vi "Flatten Value.vi"(8 "Error In":errorcluster, 11 "2D String In":refnum<class "2D String.lvclass">) -> (0 "Error Out":errorcluster, 1 "Value":string, 3 "2D String Out":refnum<class "2D String.lvclass">)   [LabVIEW 2017, in "Tree API.lvlib" / "2D String.lvclass"]
doc: "Dynamic dispatch interface for flattening Tree Data classes to string."
uses:
  2D String.lvclass
  Tree Manager/Tree.lvclass
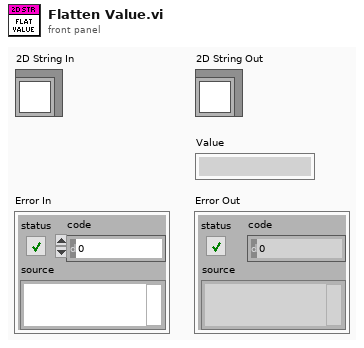
[diagram p1: front panel]
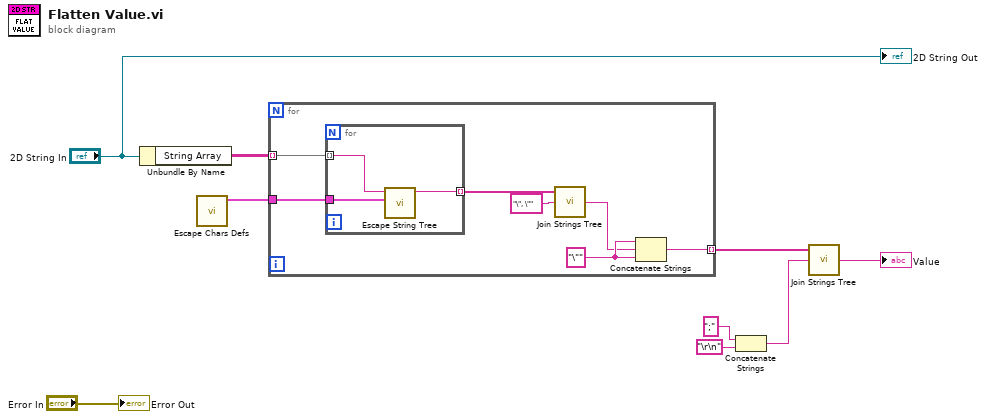
[diagram p0: block diagram]
diagram:
  n1 = Unbundle By Name("2D String In") -> ("String Array"=w9:string[][])
  n2 = call "Escape Chars Defs.vi"() -> ("Escapes"=w2:cluster{"String":string, "Escape":string}[])  [unwired: 11 in]
  n3 = for {
    tunnel: w9 -> [w15] mode=indexing
    tunnel: [w10] -> w8 mode=indexing
    tunnel: w2 -> [w16]
    w13 = "\"" ("string")
    n4 = for {
      tunnel: w16 -> [w18]
      tunnel: w15 -> [w19] mode=indexing
      tunnel: [w17] -> w11 mode=indexing
      n5 = call "Escape String Tree.vi"("Escapes"=w18, "String In"=w19) -> ("String Out"=w17:string)  [unwired: 9 in]
    }
    n6 = call "Join Strings Tree.vi"("Separator (,)"="\", \"", "Strings In"=w11) -> ("String"=w12:string)  [unwired: 1 in]
    n7 = Concatenate Strings(w13, w12, w13) -> (w10:string)
  }
  n8 = Concatenate Strings(";" ("Separator (,)"), "\r\n") -> (w4:string)
  n9 = call "Join Strings Tree.vi"("Separator (,)"=w4, "Strings In"=w8) -> ("String"=→"Value":string)  [unwired: 1 in]
  "2D String Out" <- "2D String In"
  "Error Out" <- "Error In"
